vi "430_GPIB_Query.vi"(0 "GPIB (In)":cluster{"GPIB address":i16, "GPIB bus":i16}={"GPIB address"=15, "GPIB bus"=0}, 1 "Input query":string, 2 "error in":T1) -> (3 "GPIB (Out)":cluster{"GPIB address":i16, "GPIB bus":i16}={"GPIB address"=15, "GPIB bus"=0}, 4 "Bytes returned":i32, 5 "Return string":string, 6 "error out":T1)   [LabVIEW 2018]
doc: "Implements a GPIB query given the GPIB bus information and the input query string.\n\nMultiple serial polls are performed as required after sending the query request in order to determine when bit 4 (GPIB MESSAGE AVAILABLE) is set indicating return data is available. Instruments must support the IEEE 488.2 spec for the serial poll byte for this VI to work correctly.\n\nThe response timeout setting (internal to VI) limits the amount of time the VI will wait for bit 4 to be set by the instrument."
panel:
  out "Bytes sent":i32
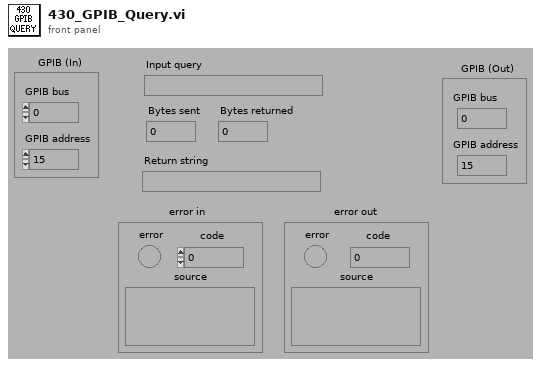
[diagram p1: front panel]
types:
  T1 = cluster{"error":bool, "code":i32, "source":string}
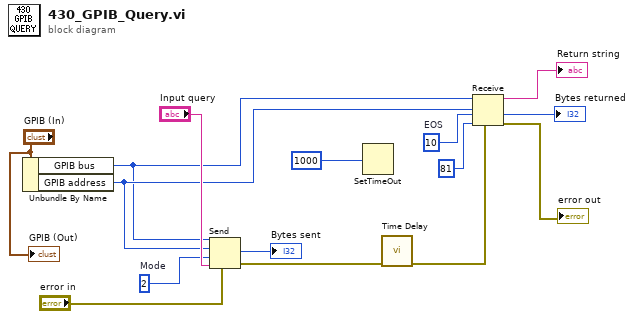
[diagram p0: block diagram]
diagram:
  w7 = i16 10  # EOS
  w6 = i16 2  # Mode
  n1 = Unbundle By Name("GPIB (In)") -> ("GPIB bus"=w4:i16, "GPIB address"=w5:i16)
  n2 = Send(0:w4, 2:w5, 3:w6, 4:"error in", 5:"Input query") -> (7:→"Bytes sent":i32, 8:w2:errorcluster)  [unwired: 1 out]
  n3 = SetTimeOut(1:1000) -> ()  [unwired: 1 out]
  n4 = call "Time Delay"("error in (no error)"=w2) -> ("error out"=w1:errorcluster)  [unwired: 10 in]
  n5 = Receive(4:w1, 6:81, 7:w7, 8:w5, 9:w4) -> (0:→"error out":errorcluster, 1:→"Bytes returned":i32, 3:→"Return string":string)  [unwired: 1 out]
  "GPIB (Out)" <- "GPIB (In)"
